vi "Alignment_2.vi"() -> ()   [LabVIEW 2011]
uses:
  Controls/LDA_Beam_Cluster.ctl
  Controls/Tunnel_Coordinates.ctl
  Controls/User_Specific_mode.ctl
  Gen Trav/Trav_mode.ctl
  Globals/Trav_pos_global.vi
panel:
  out "Beam Data":T1={"Vg1 (Green 1 dir. vect.)"=[0.059117350659853476, -0.996541267827751, 0.05840068807144843], "Vg2  (Green 2 dir. vect.)"=[-0.05232536310393669, -0.9971561380468801, -0.054237373935992664], "Vb1 (Blue 1 dir. vect.)"=[-0.052923229613528855, -0.9969242065933935, 0.057803616456121795], "Vb2 (Blue 1 dir. vect.)"=[0.05971521716944564, -0.9967731992812374, -0.05364030232066602], "Porb (Orb XYZ posn. forced coplanar)"=[2201.0738225655555, -1199.3737231995547, 269.758310600838], "Porb (Orb XYZ posn. - allow skew)"=[2200.796256301178, -1199.3740953152687, 270.0329332816893], "Orb posn. uncertainty, +/- dx, dy, dz"=[0.13878313218879157, 0.00018605785703584843, 0.13731134042564008], "Vp (Actual Probe dir. vect)"=[0.003406702197773746, -0.9999920168246164, 0.0020882210543692924], "Yaw (deg)"=89.80480953887573, "Pitch (deg)"=0.11964634006213794, "In-Plane Roll (deg)"=45.305328966424156, "Beam Half Angle (deg)"=4.544091484248422, "B1 Close P11"=[0.0, 0.0, 0.0], "B1 Far P12"=[2158.01, -491.04, 229.28], "B2 Close P22"=[2158.01, -491.04, 229.28], "B2 Far P21"=[2158.01, -491.04, 229.28], "Projected Roll (deg)"=0.0, "Green Velocity Vector"=[0.0, 0.0, 0.0], "Blue Velocity Vector"=[0.0, 0.0, 0.0], "Probe is facing...."="-", "Calculation Method"=""} {"Vp (Actual Probe dir. vect)" format="%#_6f"; "Vg2  (Green 2 dir. vect.)" format="%#_6f"; "Vg1 (Green 1 dir. vect.)" format="%#_6f"}
  in  "Distance from Orb (mm)":dbl=1500.0 format="%#.3g"
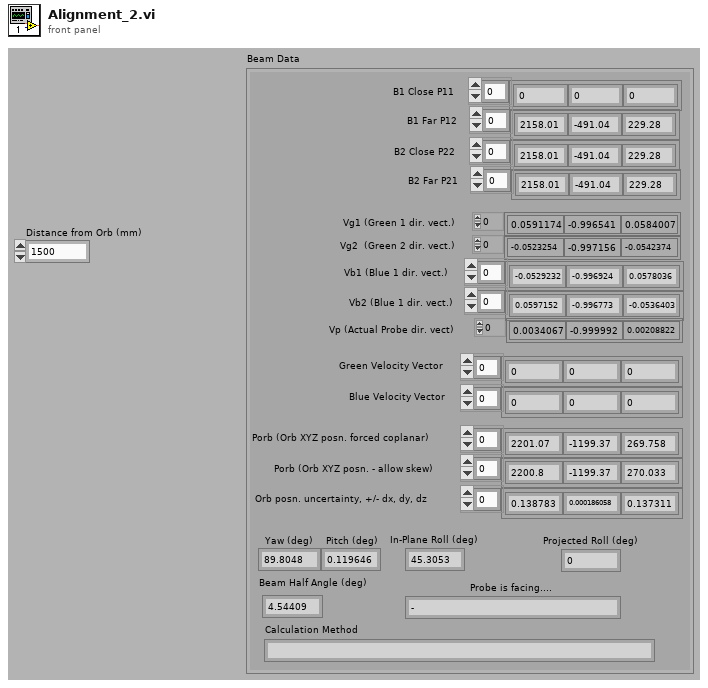
[diagram p1: front panel]
types:
  T1 = typedef "LDA_Beam_Cluster.ctl" = cluster{"Vg1 (Green 1 dir. vect.)":dbl[], "Vg2  (Green 2 dir. vect.)":dbl[], "Vb1 (Blue 1 dir. vect.)":dbl[], "Vb2 (Blue 1 dir. vect.)":dbl[], "Porb (Orb XYZ posn. forced coplanar)":dbl[], "Porb (Orb XYZ posn. - allow skew)":dbl[], "Orb posn. uncertainty, +/- dx, dy, dz":dbl[], "Vp (Actual Probe dir. vect)":dbl[], "Yaw (deg)":dbl, "Pitch (deg)":dbl, "In-Plane Roll (deg)":dbl, "Beam Half Angle (deg)":dbl, "B1 Close P11":dbl[], "B1 Far P12":dbl[], "B2 Close P22":dbl[], "B2 Far P21":dbl[], "Projected Roll (deg)":dbl, "Green Velocity Vector":dbl[], "Blue Velocity Vector":dbl[], "Probe is facing....":string, "Calculation Method":string}
  T2 = typedef "Tunnel_Coordinates.ctl" = enum16{"Work in Tunnel Coordinates", "Work in Model Coordinates"}
  T3 = enum16{"Load setup from excel file", "Save setup to excel file"}
  T4 = typedef "User_Specific_mode.ctl" = enum16{"Check VI only", "Run VI"}
  T5 = typedef "Trav_mode.ctl" = enum16{"Move traverse", "Read traverse position", "Teach Position"}
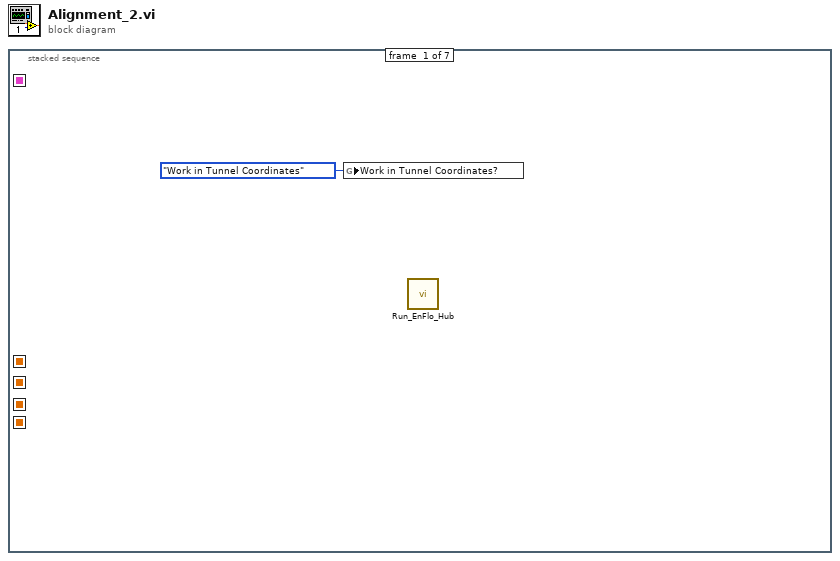
[diagram p0: block diagram]
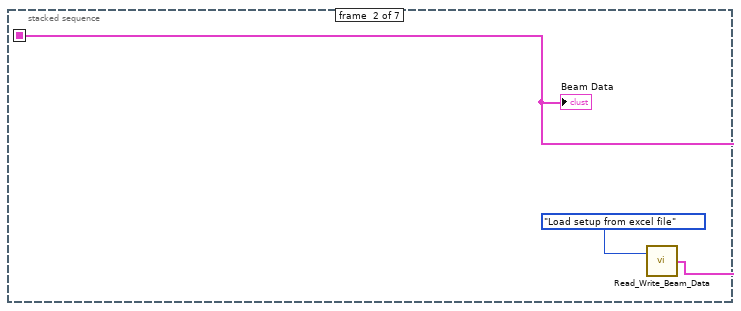
[diagram p2: hidden frame]
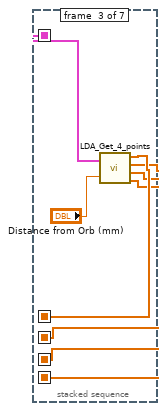
[diagram p3: hidden frame]
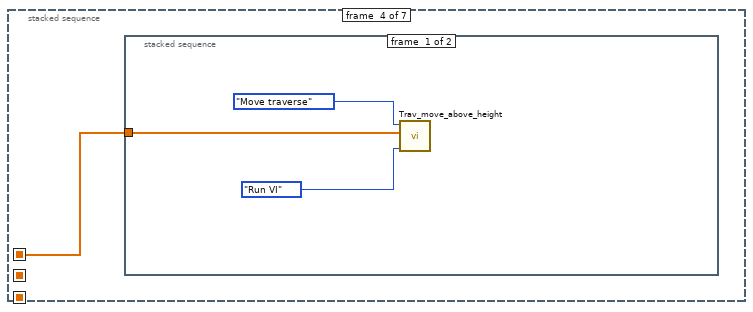
[diagram p4: hidden frame]
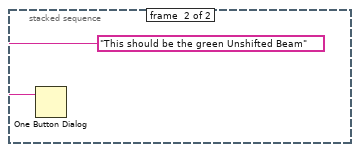
[diagram p5: hidden frame]
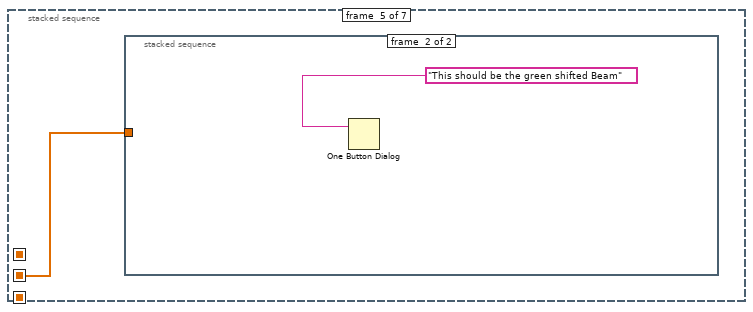
[diagram p6: hidden frame]
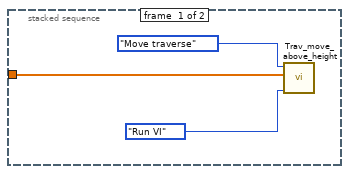
[diagram p7: hidden frame]
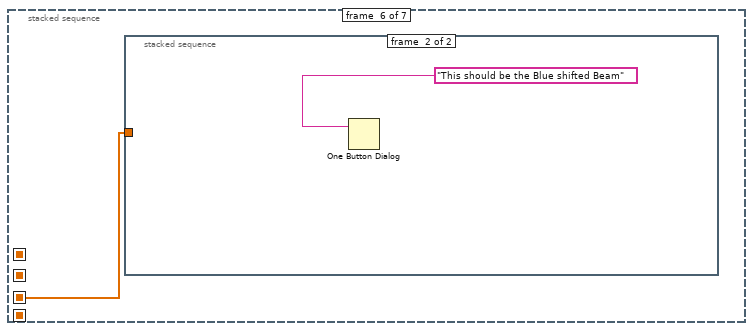
[diagram p8: hidden frame]
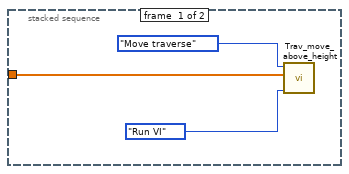
[diagram p9: hidden frame]
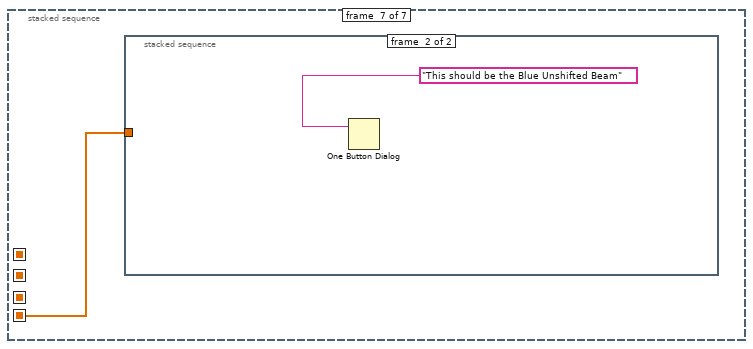
[diagram p10: hidden frame]
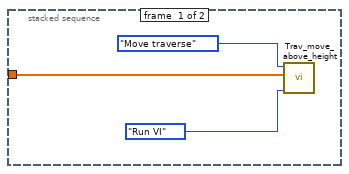
[diagram p11: hidden frame]
diagram:
  n1 = stacked-sequence {
    seq-local: [_ w2 _ _ _ _ _] -> [_ _ w9 _ _ _ _]
    seq-local: [_ _ w7 _ _ _ _] -> [_ _ _ w10 _ _ _]
    seq-local: [_ _ w6 _ _ _ _] -> [_ _ _ _ w15 _ _]
    seq-local: [_ _ w5 _ _ _ _] -> [_ _ _ _ _ w20 _]
    seq-local: [_ _ w4 _ _ _ _] -> [_ _ _ _ _ _ w25]
    frame #0 {
      n2 = global write "Trav_pos_global.vi" "Work in Tunnel Coordinates?"(Tunnel_Coordinates."Work in Tunnel Coordinates" ("Work in Tunnel Coordinates?")) -> ()
      n3 = call "Run_EnFlo_Hub.vi"() -> ()  [unwired: 8 in]
    }
    frame #1 {
      n4 = call "Read_Write_Beam_Data.vi"("Mode"=T3."Load setup from excel file") -> ("Beam Data Out"=w2:T1)  [unwired: 1 in]
      "Beam Data" <- w2
    }
    frame #2 {
      n5 = call "LDA_Get_4_points.vi"("Beam Data"=w9, "L, Probe-Normal Distance"="Distance from Orb (mm)") -> ("Pg1"=w7:dbl[], "Pg2"=w6:dbl[], "Pb1"=w5:dbl[], "Pb2"=w4:dbl[])
    }
    frame #3 {
      n6 = stacked-sequence {
        tunnel: w10 -> [w11 _]
        frame #0 {
          n7 = call "Trav_move_above_height.vi"("Simulate/Run"=User_Specific_mode."Run VI", "New Position"=w11, "Mode"=Trav_mode."Move traverse") -> ()  [unwired: 7 in, 2 out]
        }
        frame #1 {
          n8 = One Button Dialog(message="This should be the green Unshifted Beam") -> ()  [unwired: 1 in, 1 out]
        }
      }
    }
    frame #4 {
      n9 = stacked-sequence {
        tunnel: w15 -> [w16 _]
        frame #0 {
          n10 = call "Trav_move_above_height.vi"("Simulate/Run"=User_Specific_mode."Run VI", "New Position"=w16, "Mode"=Trav_mode."Move traverse") -> ()  [unwired: 7 in, 2 out]
        }
        frame #1 {
          n11 = One Button Dialog(message="This should be the green shifted Beam") -> ()  [unwired: 1 in, 1 out]
        }
      }
    }
    frame #5 {
      n12 = stacked-sequence {
        tunnel: w20 -> [w21 _]
        frame #0 {
          n13 = call "Trav_move_above_height.vi"("Simulate/Run"=User_Specific_mode."Run VI", "New Position"=w21, "Mode"=Trav_mode."Move traverse") -> ()  [unwired: 7 in, 2 out]
        }
        frame #1 {
          n14 = One Button Dialog(message="This should be the Blue shifted Beam") -> ()  [unwired: 1 in, 1 out]
        }
      }
    }
    frame #6 {
      n15 = stacked-sequence {
        tunnel: w25 -> [w26 _]
        frame #0 {
          n16 = call "Trav_move_above_height.vi"("Simulate/Run"=User_Specific_mode."Run VI", "New Position"=w26, "Mode"=Trav_mode."Move traverse") -> ()  [unwired: 7 in, 2 out]
        }
        frame #1 {
          n17 = One Button Dialog(message="This should be the Blue Unshifted Beam") -> ()  [unwired: 1 in, 1 out]
        }
      }
    }
  }
